vi "MK_Serial Setup.vi"() -> (3 "Handle":u32)   [LabVIEW 2014]
panel:
  in  "Flow Control":u16(ring) items=["None"=0, "RTS-CTS"=256, "DTR-DSR"=512, "XOn-XOff"=1024]
  in  "Word Length":u8(ring)=8 items=["FT_BITS_7"=7, "FT_BITS_8"=8]
  in  "Stop Bits":u8(ring) items=["FT_STOP_BITS_1"=0, "FT_STOP_BITS_2"=2]
  in  "Parity":u8(ring) items=["FT_PARITY_NONE", "FT_PARITY_ODD", "FT_PARITY_EVEN", "FT_PARITY_MARK", "FT_PARITY_SPACE"]
  in  "Baud Rate":u32=9600
  in  "Device Index":u32
  out "Device Description":string
  # "Inputs"
  # "Outputs"
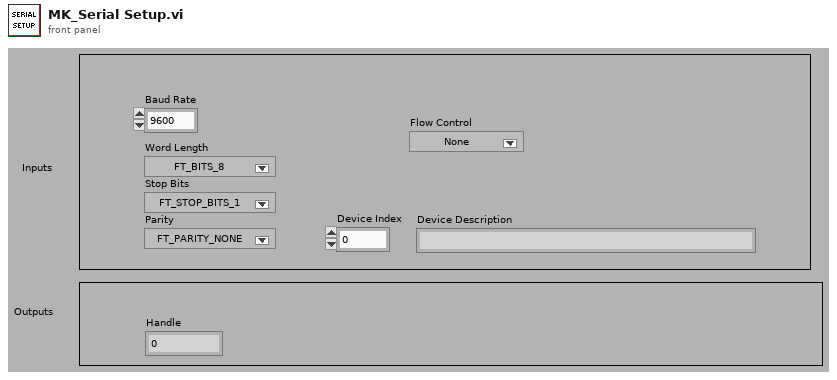
[diagram p1: front panel]
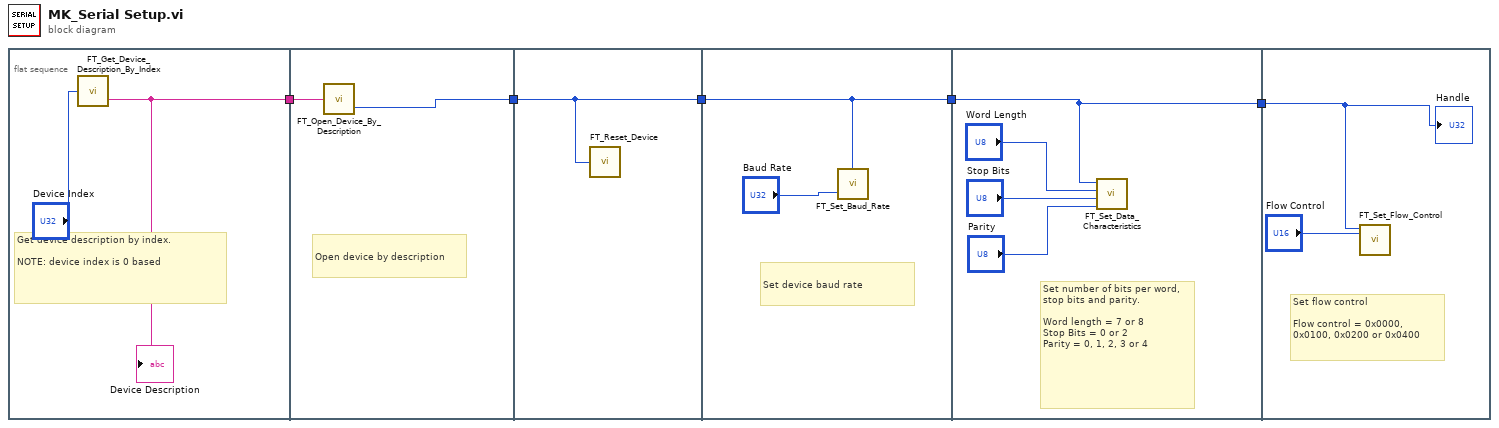
[diagram p0: block diagram]
diagram:
  n1 = flat-sequence {
    tunnel: [w7] -> w5
    tunnel: [w9] -> w4
    tunnel: w5 -> [w8]
    tunnel: w4 -> [w10]
    tunnel: [w10] -> w3
    tunnel: w3 -> [w12]
    tunnel: [w12] -> w2
    tunnel: w2 -> [w13]
    tunnel: [w13] -> w1
    tunnel: w1 -> [w17]
    frame #0 {
      # "Get device description by index.\n\nNOTE: device index is 0 based"
      n2 = call "FT_Get_Device_Description_By_Index.vi"("Device Index"="Device Index") -> ("Device Description"=w7:string)  [unwired: 1 out]
      "Device Description" <- w7
    }
    frame #1 {
      # "Open device by description"
      n3 = call "FT_Open_Device_By_Description.vi"("Device Description"=w8) -> ("Handle"=w9:u32)  [unwired: 1 out]
    }
    frame #2 {
      n4 = call "FT_Reset_Device.vi"("Handle"=w10) -> ()  [unwired: 1 out]
    }
    frame #3 {
      # "Set device baud rate"
      n5 = call "FT_Set_Baud_Rate.vi"("Baud Rate"="Baud Rate", "Handle"=w12) -> ()  [unwired: 1 out]
    }
    frame #4 {
      # "Set number of bits per word, stop bits and parity.\n\nWord length = 7 or 8\nStop Bits = 0 or 2\nParity = 0, 1, 2, 3 or 4"
      n6 = call "FT_Set_Data_Characteristics.vi"("Parity"="Parity", "Stop Bits"="Stop Bits", "Word Length"="Word Length", "Handle"=w13) -> ()  [unwired: 1 out]
    }
    frame #5 {
      # "Set flow control\n\nFlow control = 0x0000, 0x0100, 0x0200 or 0x0400"
      n7 = call "FT_Set_Flow_Control.vi"("Flow Control"="Flow Control", "Handle"=w17) -> ()  [unwired: 2 in, 1 out]
      "Handle" <- w17
    }
  }
